vi "CALC_MARK_X.vi"(0 "VISA IN":refnum<visa-resource-name>, 1 "Marker number":i32, 2 "X-axis Position":i32, 5 "error in":errorcluster, 7 "Channel":i32) -> (14 "VISA Out":refnum<visa-resource-name>, 19 "error out":errorcluster)   [LabVIEW 2018, in "PNA-X.lvlib"]
doc: "CALCulate<cnum>:MARKer<mkr>:X <num> \n(Read-Write) Sets the marker's X-axis value (frequency, power, or time). If the marker is set as delta, \nthe SET and QUERY data is relative to the reference marker. \nSee Critical Note \nParameters \n<cnum> Channel number of the measurement. There must be a selected measurement \non that channel. If unspecified, <cnum> is set to 1. \n<mkr> Any marker number from 1 to 10; if unspecified, value is set to 1. \n<num> Any X-axis position within the measurement span of the marker. \nNote: This command will accept MIN or MAX instead of a numeric \nparameter. See SCPI Syntax for more information. \nExamples CALC:MARK:X 100Mhz \ncalculate2:marker8:x maximum \nQuery Syntax CALCulate<cnum>:MARKer<mkr>:X? \nReturn Type Numeric \nDefault First Marker turns ON in the middle of the X-axis span. Subsequent markers \nturn ON at the position of the active marker. \n1542"
uses:
  PNA-X.lvlib
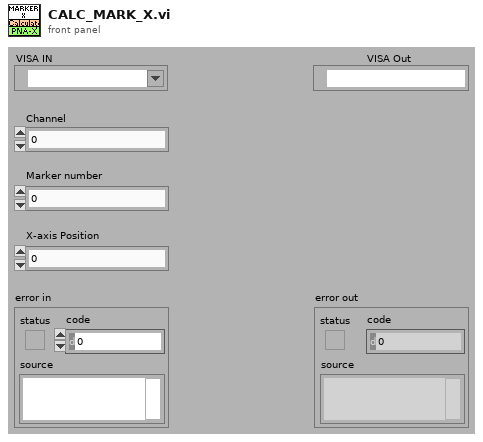
[diagram p1: front panel]
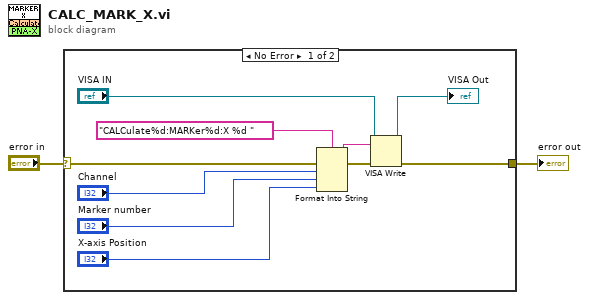
[diagram p0: block diagram]
diagram:
  n1 = case shown="No Error" "error in" {
    selector: "error in" -> [w12 w13]
    tunnel: [w7 w13] -> w1
    frame No Error {
      n2 = Format Into String(format string="CALCulate%d:MARKer%d:X %d " ("Cmdline"), error in=w12, "Channel", "Marker number", "X-axis Position") -> (resulting string=w10:string, error out=w11:errorcluster)  [unwired: 1 in]
      n3 = VISA Write(VISA resource name="VISA IN", write buffer=w10, error in (no error)=w11) -> (VISA resource name out=→"VISA Out":refnum<visa-resource-name>, error out=w7:errorcluster)  [unwired: 1 out]
    }
    frame Error {
    }
  }
  "error out" <- w1
